vi "CCD Exposure Indicator.vi"(0 "ExpTime":dbl=4.0 format="%.2f") -> ()   [LabVIEW 2025]
doc: "Author: Scott Hannahs <sth@magnet.fsu.edu>\n\nThis software is licensed for use under the “MIT License\"\nCopyright (c) 2025 Scott Hannahs, sth@sth@magnet.sthnet.net\n\nPermission is hereby granted, free of charge, to any person obtaining a copy of this software and associated documentation files (the \"Software\"), to deal in the Software without restriction, including without limitation the rights to use, copy, modify, merge, publish, distribute, sublicense, and/or sell copies of the Software, and to permit persons to whom the Software is furnished to do so, subject to the following conditions: The above copyright notice and this permission notice shall be included in all copies or substantial portions of the Software.\n\nTHE SOFTWARE IS PROVIDED \"AS IS\", WITHOUT WARRANTY OF ANY KIND, EXPRESS OR IMPLIED, INCLUDING BUT NOT LIMITED TO THE WARRANTIES OF MERCHANTABILITY, FITNESS FOR A PARTICULAR PURPOSE AND NONINFRINGEMENT. IN NO EVENT SHALL THE AUTHORS OR COPYRIGHT HOLDERS BE LIABLE FOR ANY CLAIM, DAMAGES OR OTHER LIABILITY, WHETHER IN AN ACTION OF CONTRACT, TORT OR OTHERWISE, ARISING FROM, OUT OF OR IN CONNECTION WITH THE SOFTWARE OR THE USE OR OTHER DEALINGS IN THE SOFTWARE."
uses:
  Globals and TypeDefs/Global Varibal Control.vi
  Globals and TypeDefs/gGeneral.vi
  Globals and TypeDefs/gHField.vi
panel:
  out "x-y":u32
  out "Exp flash":string caption="Exposure"
  out "Exposure":dbl(slide)=0.133 scale=0.0..10.0 scale format="%.1f"
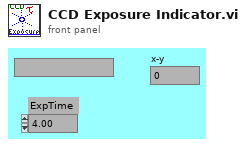
[diagram p1: front panel]
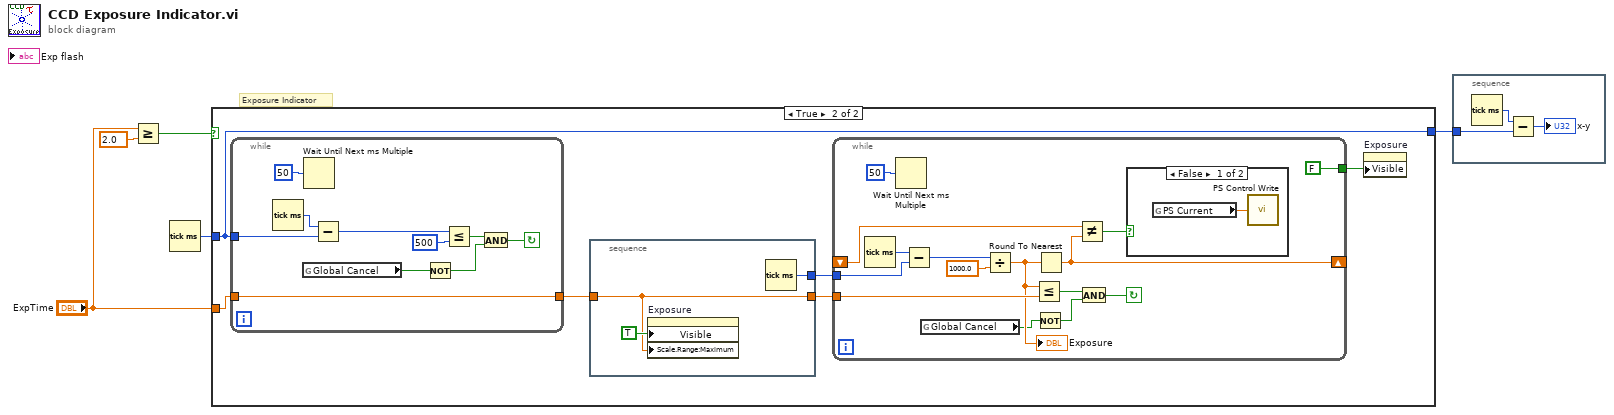
[diagram p0: block diagram]
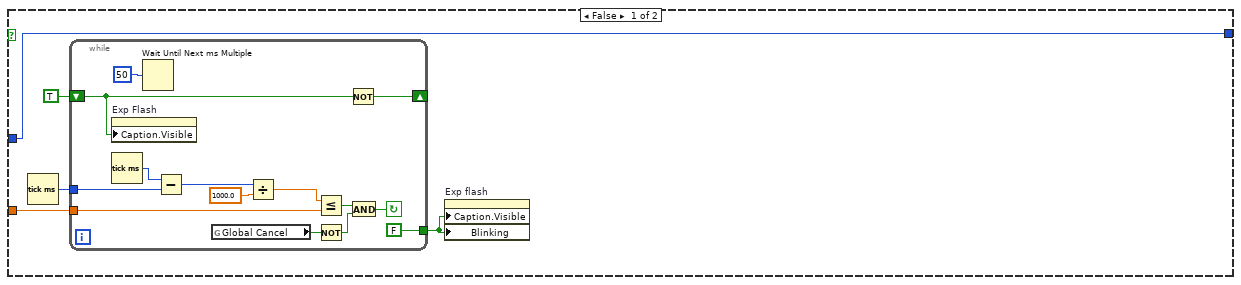
[diagram p2: hidden frame]
diagram:
  # "Exposure Indicator"
  n1 = Greater Or Equal?(x="ExpTime", y=2.0) -> (x >= y?=w5:bool)
  n2 = Tick Count (ms)() -> (millisecond timer value=w2:u32)
  n3 = case shown="True" w5 {
    tunnel: "ExpTime" -> [w7 w26]
    tunnel: [w6 w27] -> w1
    tunnel: w2 -> [w6 w27]
    frame False {
      n4 = Tick Count (ms)() -> (millisecond timer value=w10:u32)
      n5 = while {
        shift-left: TRUE ("Visible") -> [w15]
        shift-right: [w16] -> _
        tunnel: [FALSE ("Visible")] -> w9
        tunnel: w7 -> [w17]
        tunnel: w10 -> [w21]
        stop <- w12 continue-if-true
        n6 = property on="Exp Flash" class="Str"("Caption.Visible"=w15) -> ()  [unwired: 2 in, 2 out]
        n7 = Tick Count (ms)() -> (millisecond timer value=w23:u32)
        n8 = Wait Until Next ms Multiple(millisecond multiple=u32 50) -> ()  [unwired: 1 out]
        n9 = Subtract(x=w23, y=w21) -> (x-y=w22:u32)
        n10 = global read "Global Varibal Control.vi" "Global Cancel"() -> (w11:bool)
        n11 = Divide(x=w22, y=1000.0) -> (x/y=w18:dbl)
        n12 = Less Or Equal?(x=w18, y=w17) -> (x <= y?=w13:bool)
        n13 = Not(x=w11) -> (.not. x?=w14:bool)
        n14 = Not(x=w15) -> (.not. x?=w16:bool)
        n15 = And(x=w13, y=w14) -> (x .and. y?=w12:bool)
      }
      n16 = property on="Exp flash" class="Str"("Caption.Visible"=w9, "Blinking"=w9) -> ()  [unwired: 2 in, 2 out]
    }
    frame True {
      n17 = while {
        tunnel: [w49] -> w25
        tunnel: w26 -> [w49]
        tunnel: w27 -> [w48]
        stop <- w52 continue-if-true
        n18 = Tick Count (ms)() -> (millisecond timer value=w56:u32)
        n19 = global read "gGeneral.vi" "Global Cancel"() -> (w47:bool)
        n20 = Wait Until Next ms Multiple(millisecond multiple=u32 50) -> ()  [unwired: 1 out]
        n21 = Subtract(x=w56, y=w48) -> (x-y=w51:u32)
        n22 = Not(x=w47) -> (.not. x?=w54:bool)
        n23 = Less Or Equal?(x=w51, y=u32 500 ("millisecond multiple")) -> (x <= y?=w53:bool)
        n24 = And(x=w53, y=w54) -> (x .and. y?=w52:bool)
      }
      n25 = stacked-sequence {
        tunnel: [w58] -> w30
        tunnel: w25 -> [w57]
        tunnel: [w57] -> w29
        frame #0 {
          n26 = property on="Exposure" class="Slide (strict)"("Visible"=TRUE, "Scale.Range:Maximum"=w57) -> ()  [unwired: 2 in, 2 out]
          n27 = Tick Count (ms)() -> (millisecond timer value=w58:u32)
        }
      }
      n28 = while {
        shift-left: _ -> [w35]
        shift-right: [w32] -> _
        tunnel: [FALSE ("Visible")] -> w28
        tunnel: w29 -> [w41]
        tunnel: w30 -> [w42]
        stop <- w37 continue-if-true
        n29 = Tick Count (ms)() -> (millisecond timer value=w44:u32)
        n30 = Wait Until Next ms Multiple(millisecond multiple=u32 50) -> ()  [unwired: 1 out]
        n31 = Subtract(x=w44, y=w42) -> (x-y=w43:u32)
        n32 = global read "gGeneral.vi" "Global Cancel"() -> (w31:bool)
        n33 = Divide(x=w43, y=1000.0) -> (x/y=w33:dbl)
        "Exposure" <- w33
        n34 = Less Or Equal?(x=w33, y=w41) -> (x <= y?=w38:bool)
        n35 = Not(x=w31) -> (.not. x?=w39:bool)
        n36 = Round To Nearest(number=w33) -> (nearest integer value=w32:dbl)
        n37 = Not Equal?(x=w35, y=w32) -> (x != y?=w34:bool)
        n38 = And(x=w38, y=w39) -> (x .and. y?=w37:bool)
        n39 = case shown="False" w34 {
          frame False {
            n40 = global read "gHField.vi" "PS Current"() -> (w46:dbl)
            n41 = call "PS Control Write.vi"("Setpoint"=w46) -> ()  [unwired: 13 in, 2 out]
          }
          frame True {
          }
        }
      }
      n42 = property on="Exposure" class="Slide (strict)"("Visible"=w28) -> ()  [unwired: 2 in, 2 out]
    }
  }
  n43 = stacked-sequence {
    tunnel: w1 -> [w62]
    frame #0 {
      n44 = Tick Count (ms)() -> (millisecond timer value=w61:u32)
      n45 = Subtract(x=w61, y=w62) -> (x-y=→"x-y":u32)
    }
  }
